vi "Functional Test.vi"() -> ()   [LabVIEW 2017]
uses:
  <vilib>/Instr/_visa.llb/VISA Configure Serial Port (Instr).vi
panel:
  out "read buffer":string
  in  "Send Command":bool
  in  "Command":string
  out "Write length":i32
  in  "Time (s)":dbl
  out "Read length":i32
  in  "Baud Rate":u32
  out "Read":string[](array[string])
  in  "VISA resource name":refnum<visa-resource-name>
  out "Error Out":errorcluster
  in  "Error In":errorcluster
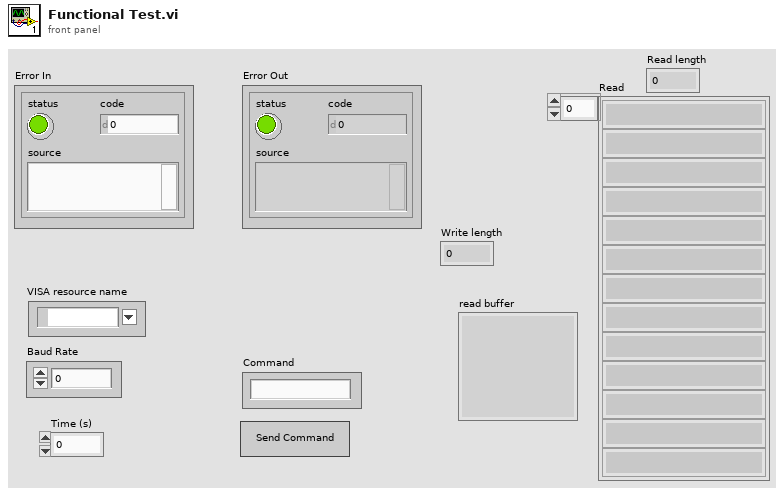
[diagram p1: front panel]
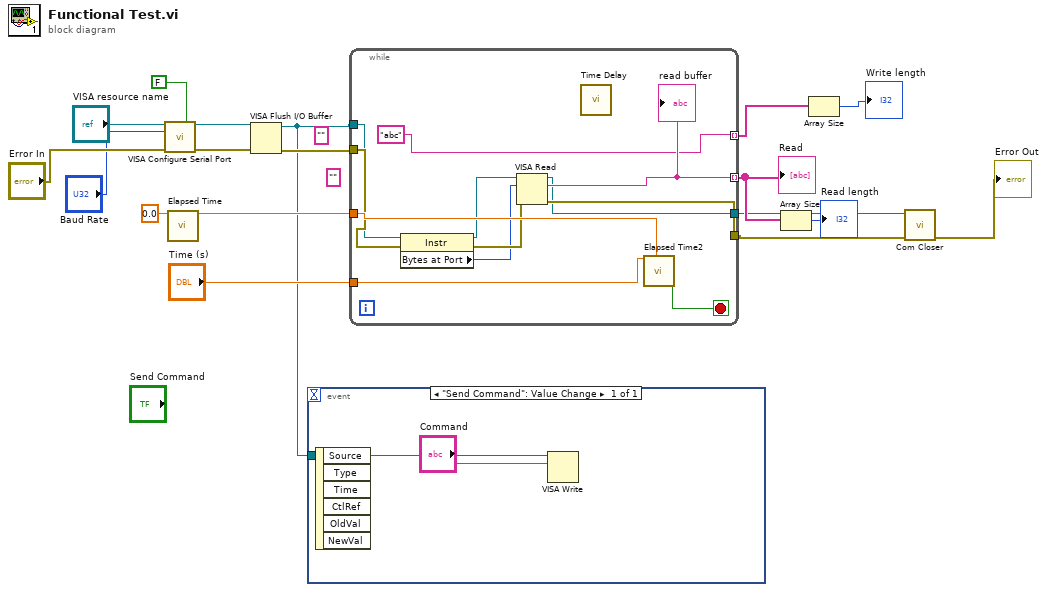
[diagram p0: block diagram]
diagram:
  (unwired) ""
  (unwired) ""
  n1 = call-poly "VISA Configure Serial Port"("VISA resource name"="VISA resource name", "Enable Termination\nChar (T)"=FALSE ("Enable Termination\nChar (T)"), "baud rate (9600)"="Baud Rate", "error in (no error)"="Error In") -> ("VISA resource name out"=w6:refnum<visa-resource-name>, "error out"=w8:errorcluster)  [unwired: 10 in]
  n2 = call "Elapsed Time"("Time Target (s)"=0.0) -> ("Present (s)"=w18:dbl)  [unwired: 11 in, 7 out]
  n3 = VISA Flush I/O Buffer(VISA resource name=w6, error in (no error)=w8) -> (VISA resource name out=w2:refnum<visa-resource-name>, error out=w7:errorcluster)  [unwired: 1 in]
  n4 = event shown="[0] \"Send Command\": Value Change" {
    selector: _ -> [_]
    dyn-events: _ -> [_]
    timeout: _ -> [_]
    tunnel: w2 -> [w19]
    event "Send Command": Value Change {
      n5 = event-data() -> ()  [unwired: 1 in, 6 out]
      n6 = VISA Write(VISA resource name=w19, write buffer="Command") -> ()  [unwired: 1 in, 3 out]
    }
  }
  n7 = while {
    tunnel: w18 -> [w31]
    tunnel: w2 -> [w29]
    tunnel: w7 -> [w30]
    tunnel: "Time (s)" -> [w26]
    tunnel: [w25] -> w13 mode=indexing
    tunnel: ["abc" ("write buffer")] -> w9 mode=indexing
    tunnel: [w23] -> w5
    tunnel: [w22] -> w3
    stop <- w32 stop-if-true
    n8 = property class="Instr"(reference=w29, error in=w30) -> (reference out=w28:refnum<visa-resource-name>, error out=w27:errorcluster, "Bytes at Port"=w21:u32)
    n9 = VISA Read(VISA resource name=w28, byte count=w21, error in (no error)=w27) -> (VISA resource name out=w22:refnum<visa-resource-name>, read buffer=w25:string, error out=w23:errorcluster)  [unwired: 1 out]
    "read buffer" <- w25
    n10 = call "Time Delay"() -> ()  [unwired: 11 in, 1 out]
    n11 = call "Elapsed Time2"("Time Target (s)"=w26, "Set Start Time (s)"=w31) -> ("Time has Elapsed"=w32:bool)  [unwired: 10 in, 7 out]
  }
  "Read" <- w13
  n12 = Array Size(array=w13) -> (size(s)=→"Read length":i32)
  n13 = Array Size(array=w9) -> (size(s)=→"Write length":i32)
  n14 = call "Com Closer.vi"("Error In"=w5, "VISA resource name"=w3) -> ("Error Out"=→"Error Out":errorcluster)  [unwired: 9 in]
